vi "Get Next State.vi"(8 "Error In":errorcluster, 11 "Array Input":T1[](array[typedef])) -> (0 "Error Out":errorcluster, 1 "Current State":T1=enum."User Login", 3 "Remaining States":T1[](array[typedef]))   [LabVIEW 2014]
doc: "The VI gets the new state from states array.\nDeletes the new state from states array.\nIf array is empty, outputs idle state."
uses:
  Controls/MainEnum.ctl
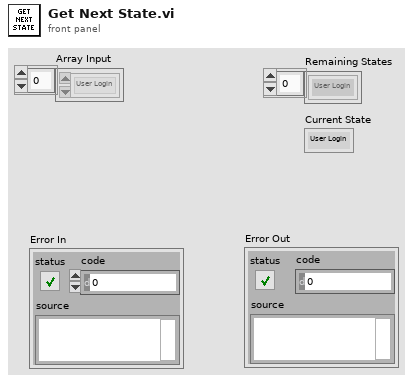
[diagram p1: front panel]
types:
  T1 = typedef "MainEnum.ctl" = enum16{"LOAD CALIBRATION DATA", "Pre Initialize", "Quality INS", "Idle", "User Login", "Initialize", "Update Tabs", "Data Initialize", "Exit", "Update Front Panel", "Vision Position", "Slider Positioning", "System Dispense", "Return to orig", "Vision Quality", "System Init", "Emergency Stop", "Data Update: Global", "Actuators ON/OFF", "Paste Expired", "Syringe Replacement", "System Dispense0", "ReturnOrig0", "Syringe Init", "Vision Position2", "Alarm", "Door Sensor", "Vision Quality 2", "Gripper", "Positioning Error0", "Maintenance", "QualDispense0", "QualDispense", "Positioning Error", "Start Test", "Slider Positioning Old", "Beforee", "System Dispense0new", "Moving Quality", "Return from Qual", "Positioning Error 600+"}
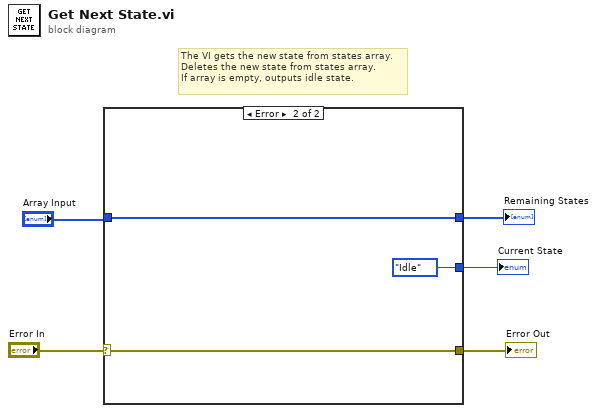
[diagram p0: block diagram]
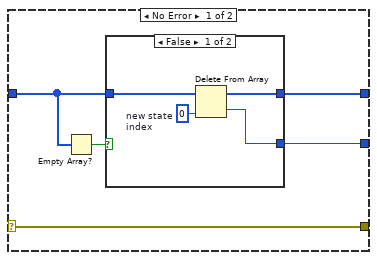
[diagram p2: hidden frame]
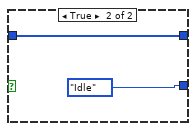
[diagram p3: hidden frame]
diagram:
  # "The VI gets the new state from states array.\nDeletes the new state from states array.\nIf array is empty, outputs idle state."
  n1 = case shown="Error" "Error In" {
    selector: "Error In" -> [w6 w19]
    tunnel: "Array Input" -> [w10 w18]
    tunnel: [w9 w18] -> w2
    tunnel: [w7 MainEnum."Idle" ("Enum")] -> w3
    tunnel: [w6 w19] -> w4
    frame No Error {
      n2 = Empty Array?(array=w10) -> (empty?=w8:bool)
      n3 = case shown="False" w8 {
        tunnel: w10 -> [w14 w16]
        tunnel: [w13 MainEnum."Idle" ("Enum")] -> w7
        tunnel: [w11 w16] -> w9
        frame False {
          w12 = 0  # new state index
          n4 = Delete From Array(array=w14, index=w12) -> (deleted portion=w13:T1, array with subset deleted=w11:T1[])  [unwired: 1 in]
        }
        frame True {
        }
      }
    }
    frame Error {
    }
  }
  "Error Out" <- w4
  "Remaining States" <- w2
  "Current State" <- w3
